vi "Get Ideal Fundamental and IMD Slopes - TOI.vi"(0 "Test Configuration in":T2={"Target Pout Per Tone (dBm)"=0.0, "Start Value"={"Power Level per Tone (dBm)"=0.0, "Center Frequency (Hz)"=0.0, "Tone Spacing (Hz)"=0.0}, "Sweep Settings"={"Mode"=enum."Power", "Sweep Delay (ms)"=0, "Power Sweep End"=-20.0, "Power Sweep Step"=-20.0, "Frequency Sweep End"=-4.0, "Frequency Sweep Step"=1.0, "Tone Spacing Sweep End"=-4.0, "Tone Spacing Sweep Step"=1.0}} {"Sweep Settings"."Tone Spacing Sweep Step" format="%#.pHz"; "Sweep Settings"."Tone Spacing Sweep End" format="%#.pHz"; "Sweep Settings"."Frequency Sweep Step" format="%#.pHz"; "Sweep Settings"."Frequency Sweep End" format="%#.pHz"; "Sweep Settings"."Power Sweep End" format="%#_6p"; "Sweep Settings"."Sweep Delay (ms)" format="%#.3p"; "Start Value"."Tone Spacing (Hz)" format="%#_6p"; "Start Value"."Center Frequency (Hz)" format="%#.3p"}, 1 "Sweep a-xis":dbl[](array[numeric]), 5 "List of Fundamental Pout":dbl[](array[numeric]), 7 "List of PINs":dbl[](array[numeric]), 9 "List of OIP3":dbl[](array[numeric]), 11 "List of IMD":dbl[](array[numeric])) -> (2 "Sweep a-xis":dbl[](array[numeric]), 3 "Fundamental and IMD Slope":cluster{dbl[], dbl[]}[](graph), 4 "Test Configuration out":T2={"Target Pout Per Tone (dBm)"=0.0, "Start Value"={"Power Level per Tone (dBm)"=0.0, "Center Frequency (Hz)"=0.0, "Tone Spacing (Hz)"=0.0}, "Sweep Settings"={"Mode"=enum."Power", "Sweep Delay (ms)"=0, "Power Sweep End"=-20.0, "Power Sweep Step"=-20.0, "Frequency Sweep End"=-4.0, "Frequency Sweep Step"=1.0, "Tone Spacing Sweep End"=-4.0, "Tone Spacing Sweep Step"=1.0}} {"Sweep Settings"."Tone Spacing Sweep Step" format="%#.pHz"; "Sweep Settings"."Tone Spacing Sweep End" format="%#.pHz"; "Sweep Settings"."Frequency Sweep Step" format="%#.pHz"; "Sweep Settings"."Frequency Sweep End" format="%#.pHz"; "Sweep Settings"."Power Sweep End" format="%#_6p"; "Sweep Settings"."Sweep Delay (ms)" format="%#.3p"; "Start Value"."Tone Spacing (Hz)" format="%#_6p"; "Start Value"."Center Frequency (Hz)" format="%#.3p"}, 6 "List of Fundamental Pout":dbl[](array[numeric]), 8 "List of PINs":dbl[](array[numeric]), 10 "List of OIP3":dbl[](array[numeric]), 14 "Results - Target Pout per Tone":T1, 15 "List of IMD":dbl[](array[numeric]))   [LabVIEW 2023]
uses:
  Controls/Test Config - TOI.ctl
  Controls/Target Pout per Tone Results Cluster - TOI.ctl
  <vilib>/Analysis/baseanly.llb/Mean (DBL).vi
  <vilib>/Analysis/NI_AALBase.lvlib
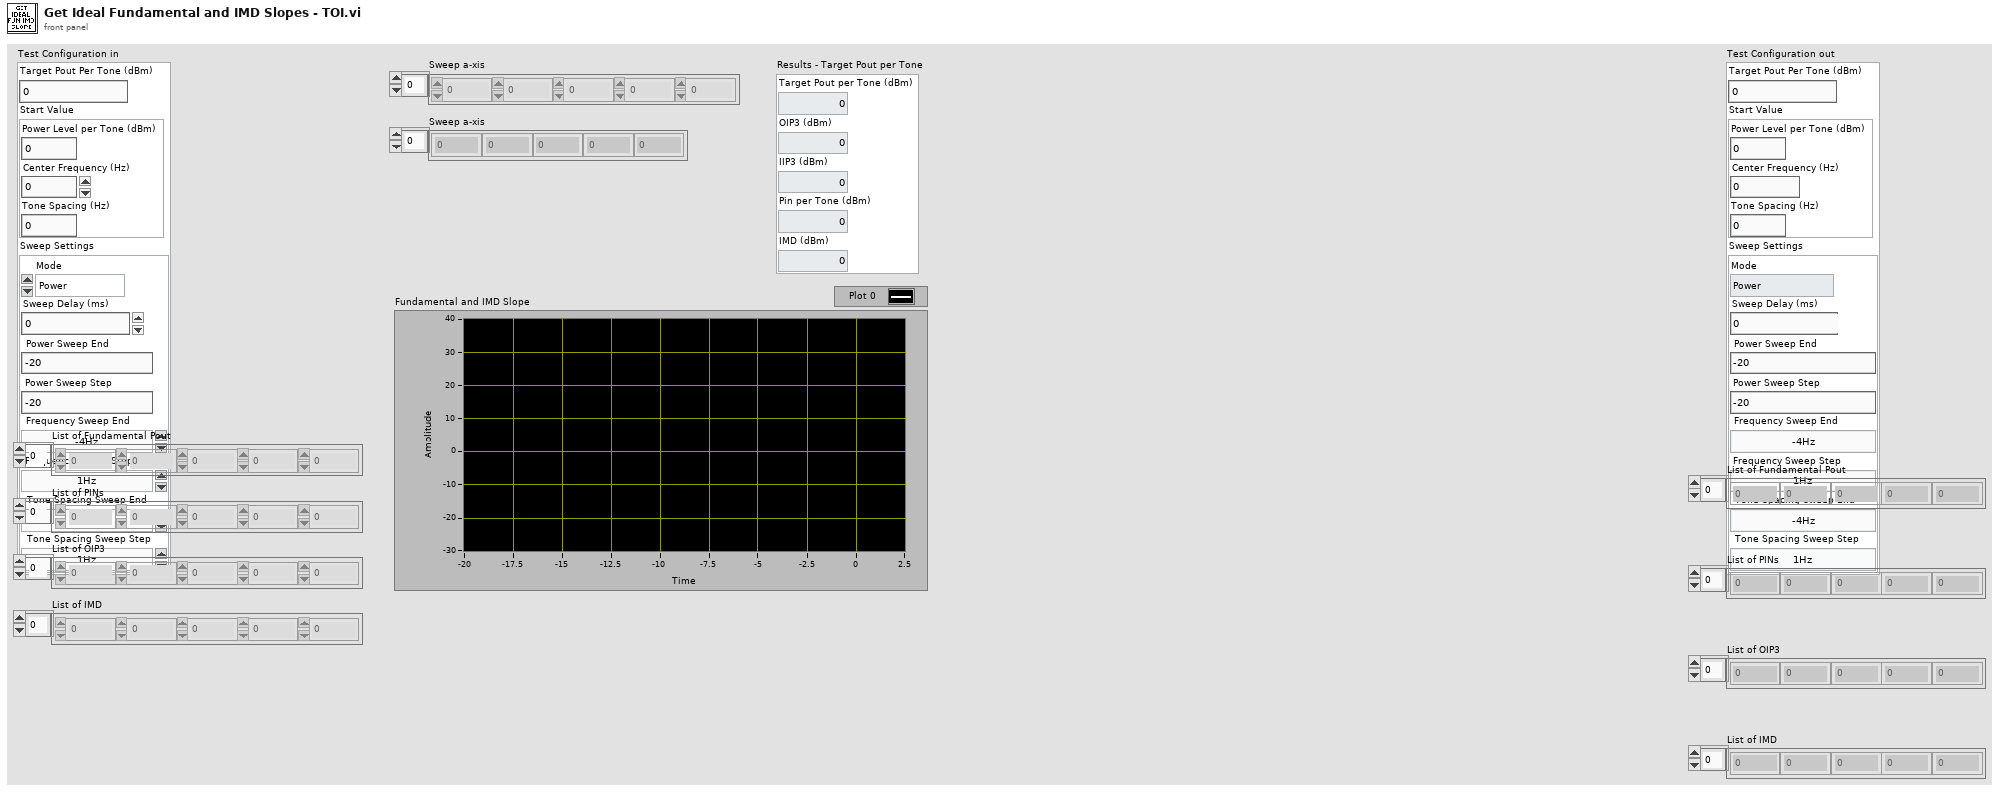
[diagram p1: front panel]
types:
  T1 = typedef "Target Pout per Tone Results Cluster - TOI.ctl" = cluster{"Target Pout per Tone (dBm)":dbl, "OIP3 (dBm)":dbl, "IIP3 (dBm)":dbl, "Pin per Tone (dBm)":dbl, "IMD (dBm)":dbl}
  T2 = typedef "Test Config - TOI.ctl" = cluster{"Target Pout Per Tone (dBm)":dbl, "Start Value":cluster{"Power Level per Tone (dBm)":dbl, "Center Frequency (Hz)":dbl, "Tone Spacing (Hz)":dbl}, "Sweep Settings":cluster{"Mode":enum16{"Power", "Frequency", "Tone Spacing"}, "Sweep Delay (ms)":u32, "Power Sweep End":dbl, "Power Sweep Step":dbl, "Frequency Sweep End":dbl, "Frequency Sweep Step":dbl, "Tone Spacing Sweep End":dbl, "Tone Spacing Sweep Step":dbl}}
  T3 = cluster{"List of PINs":dbl[], "Fundamental Slope":dbl[]}
  T4 = cluster{"List of PINs":dbl[], "IMD Slope":dbl[]}[]
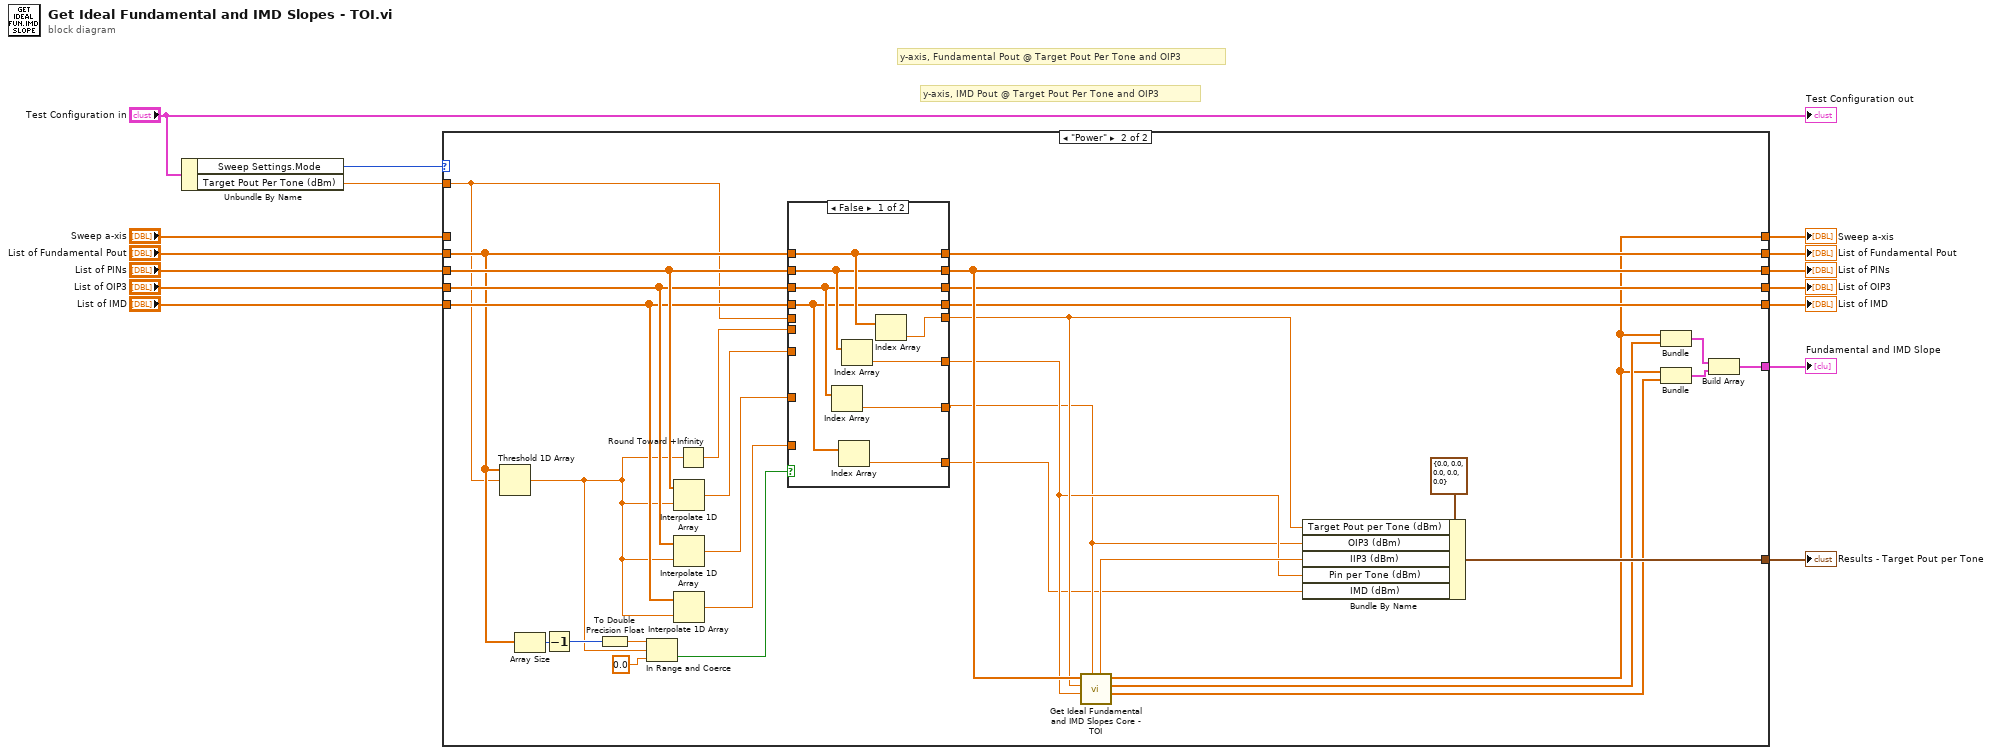
[diagram p0: block diagram]
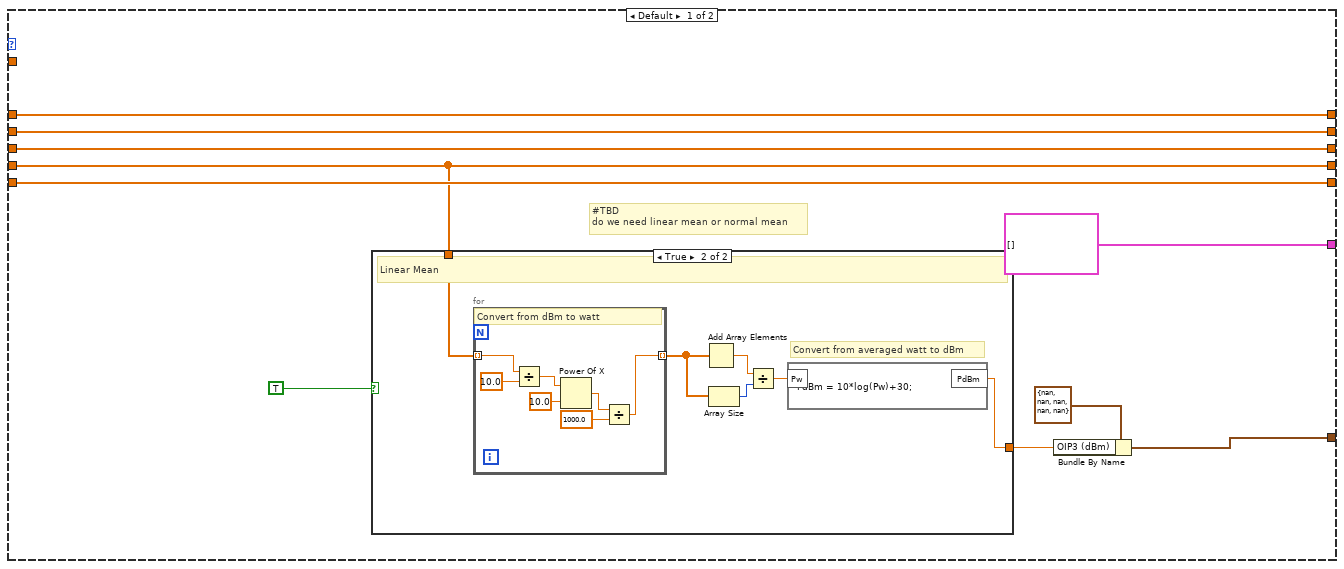
[diagram p2: hidden frame]
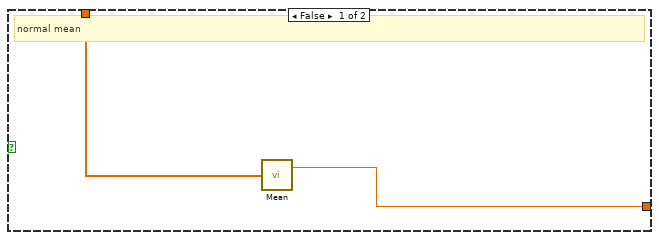
[diagram p3: hidden frame]
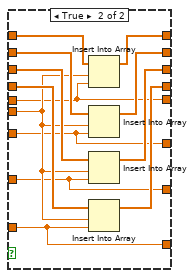
[diagram p4: hidden frame]
diagram:
  # "y-axis, IMD Pout @ Target Pout Per Tone and OIP3"
  # "y-axis, Fundamental Pout @ Target Pout Per Tone and OIP3"
  n1 = Unbundle By Name("Test Configuration in") -> ("Sweep Settings.Mode"=w7:enum16{"Power", "Frequency", "Tone Spacing"}, "Target Pout Per Tone (dBm)"=w12:dbl)
  n2 = case shown="\"Power\"" w7 {
    tunnel: [cluster{dbl[], dbl[]}[] [] w72] -> w15
    tunnel: [w19 w71] -> w13
    tunnel: w12 -> [_ w48]
    tunnel: "List of PINs" -> [w23 w67]
    tunnel: "List of Fundamental Pout" -> [w24 w49]
    tunnel: "List of OIP3" -> [w18 w66]
    tunnel: "List of IMD" -> [w22 w65]
    tunnel: "Sweep a-xis" -> [w21 _]
    tunnel: [w23 w60] -> w5
    tunnel: [w18 w59] -> w4
    tunnel: [w22 w58] -> w3
    tunnel: [w24 w61] -> w2
    tunnel: [w21 w57] -> w1
    frame Default {
      # "#TBD\ndo we need linear mean or normal mean"
      n3 = case shown="True" TRUE {
        tunnel: w18 -> [w27 w33]
        tunnel: [w26 w28] -> w17
        frame False {
          # "normal mean"
          n4 = call-poly <vilib>:"Mean.vi"("X"=w27) -> ("mean"=w26:dbl)  [unwired: 1 out]
        }
        frame True {
          # "Convert from averaged watt to dBm"
          # "Linear Mean"
          n5 = for {
            tunnel: w33 -> [w38] mode=indexing
            tunnel: [w34] -> w32 mode=indexing
            # "Convert from dBm to watt"
            n6 = Divide(x=w38, y=10.0) -> (x/y=w40:dbl)
            n7 = Power Of X(1:10.0 ("x"), 2:w40) -> (0:w36:dbl)
            n8 = Divide(x=w36, y=1000.0) -> (x/y=w34:dbl)
          }
          n9 = Add Array Elements(numeric array=w32) -> (sum=w31:dbl)
          n10 = Array Size(array=w32) -> (size(s)=w30:i32)
          n11 = Divide(x=w31, y=w30) -> (x/y=w29:dbl)
          n12 = formula code="PdBm = 10*log(Pw)+30;"("Pw"=w29) -> ("PdBm"=w28:dbl)
        }
      }
      n13 = Bundle By Name(cluster=T1 {"Target Pout per Tone (dBm)"=nan, "OIP3 (dBm)"=nan, "IIP3 (dBm)"=nan, "Pin per Tone (dBm)"=nan, "IMD (dBm)"=nan} ("Results - Target Pout per Tone"), "OIP3 (dBm)"=w17) -> (w19:T1)
    }
    frame "Power" {
      n14 = Threshold 1D Array(2:w48, 3:w49) -> (0:w46:dbl)  [unwired: 1 in]
      n15 = Array Size(array=w49) -> (size(s)=w51:i32)
      n16 = Decrement(x=w51) -> (x-1=w47:i32)
      n17 = To Double Precision Float(number=w47) -> (double precision float=w45:dbl)
      n18 = In Range and Coerce(upper limit=w45, x=w46, lower limit=0.0) -> (In Range?=w50:bool)  [unwired: 1 out]
      n19 = Interpolate 1D Array(1:w46, 2:w67) -> (0:w63:dbl)
      n20 = Interpolate 1D Array(1:w46, 2:w66) -> (0:w53:dbl)
      n21 = Interpolate 1D Array(1:w46, 2:w65) -> (0:w62:dbl)
      n22 = Round Toward +Infinity(x=w46) -> (ceil(x): smallest int >= x=w64:dbl)
      n23 = case shown="False" w50 {
        tunnel: w67 -> [w78 w93]
        tunnel: w66 -> [w76 w92]
        tunnel: w65 -> [w73 w91]
        tunnel: w64 -> [_ w86]
        tunnel: w63 -> [_ w83]
        tunnel: w53 -> [_ w82]
        tunnel: w62 -> [_ w81]
        tunnel: [w78 w90] -> w60
        tunnel: [w76 w89] -> w59
        tunnel: [w73 w88] -> w58
        tunnel: w49 -> [w80 w87]
        tunnel: w48 -> [_ w84]
        tunnel: [w80 w85] -> w61
        tunnel: [w79 w84] -> w44
        tunnel: [w77 w83] -> w43
        tunnel: [w75 w82] -> w42
        tunnel: [w74 w81] -> w41
        frame False {
          n24 = Index Array(array=w76) -> (element=w75:dbl)  [unwired: 1 in]
          n25 = Index Array(array=w73) -> (element=w74:dbl)  [unwired: 1 in]
          n26 = Index Array(array=w78) -> (element=w77:dbl)  [unwired: 1 in]
          n27 = Index Array(array=w80) -> (element=w79:dbl)  [unwired: 1 in]
        }
        frame True {
          n28 = Insert Into Array(array=w87, index=w86, new element=w84) -> (w85:dbl[])
          n29 = Insert Into Array(array=w93, index=w86, new element=w83) -> (w90:dbl[])
          n30 = Insert Into Array(array=w92, index=w86, new element=w82) -> (w89:dbl[])
          n31 = Insert Into Array(array=w91, index=w86, new element=w81) -> (w88:dbl[])
        }
      }
      n32 = call "Get Ideal Fundamental and IMD Slopes Core - TOI.vi"("OIP3"=w42, "Target Pin Per Tone (dBm)"=w43, "Target Pout Per Tone (dBm)"=w44, "List of PINs"=w60) -> ("IMD Slope"=w56:dbl[], "Fundamental Slope"=w70:dbl[], "List of PINs"=w57:dbl[], "IIP3"=w54:dbl)  [unwired: 4 in]
      n33 = Bundle By Name(cluster=T1 {"Target Pout per Tone (dBm)"=0.0, "OIP3 (dBm)"=0.0, "IIP3 (dBm)"=0.0, "Pin per Tone (dBm)"=0.0, "IMD (dBm)"=0.0} ("Results - Target Pout per Tone"), "Target Pout per Tone (dBm)"=w44, "OIP3 (dBm)"=w42, "IIP3 (dBm)"=w54, "Pin per Tone (dBm)"=w43, "IMD (dBm)"=w41) -> (w71:T1)
      n34 = Bundle("List of PINs"=w57, "Fundamental Slope"=w70) -> (w69:T3)  [unwired: 1 in]
      n35 = Bundle("List of PINs"=w57, "IMD Slope"=w56) -> (w55:cluster{"List of PINs":dbl[], "IMD Slope":dbl[]})  [unwired: 1 in]
      n36 = Build Array(w69, w55) -> (w72:T4)
    }
  }
  "Fundamental and IMD Slope" <- w15
  "Results - Target Pout per Tone" <- w13
  "List of PINs" <- w5
  "List of IMD" <- w3
  "List of OIP3" <- w4
  "List of Fundamental Pout" <- w2
  "Sweep a-xis" <- w1
  "Test Configuration out" <- "Test Configuration in"
